vi "PH_PILS.set Doors Beam Diag.vi"(0 "i ref in":refnum<vi>, 2 "Service Name":string="N/A", 5 "error in":errorcluster) -> (14 "i ref out":refnum<vi>, 19 "error out":errorcluster)   [LabVIEW 2014, in "PH_PILS.lvlib"]
doc: "This VI sets the GUI elements related to the doors at the beam Diagnostic."
uses:
  PH_PILS.lvlib
  PH_PILS.Operation Mode.ctl
  PH_Common/PH_Common.lvlib
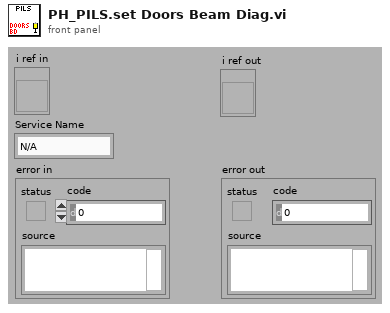
[diagram p1: front panel]
types:
  T1 = typedef "PH_PILS.lvlib/PH_PILS.Operation Mode.ctl" = enum16{"unknown", "Service", "Labor", "Search", "Shot"}
  T2 = typedef "PH_PILS.lvlib/PH_PILS.i attribute.ctl" = cluster{"Boolean":cluster{"GUI Ref":refnum<vi>, "Status":i32}[], "GUI Refs Exp. Shutters":cluster{"1":refnum<vi>, "2":refnum<vi>, "3":refnum<vi>, "4":refnum<vi>}, "Tristate2Run GUI Refs":refnum<vi>[], "EO-Likes":cluster{"GUI Ref":refnum<vi>, "Status":i32}[], "Operation Mode":cluster{"Operation Mode":T1, "GUI":cluster{"Ref State":refnum<vi>, "Ref":refnum<vi>}, "Servicemode":cluster{"Tagname":string, "Status":i32}, "Labormode":cluster{"Tagname":string, "Status":i32}, "Searchmode":cluster{"Tagname":string, "Status":i32}, "Shotmode":cluster{"Tagname":string, "Status":i32}}, "Submode":cluster{"Submode":T3, "GUI":cluster{"Ref State":refnum<vi>, "Ref":refnum<vi>}, "Submode":cluster{"Tagname":string, "Status":i32}}, "Experiment":cluster{"Experiment":enum16{"unknown", "intern", "4 (Z6)", "3", "2", "1"}, "GUI":cluster{"Ref State":refnum<vi>, "Ref":refnum<vi>}, "intern":cluster{"Tagname":string, "Status":i32}, "Exp 4":cluster{"Tagname":string, "Status":i32}, "Exp 3":cluster{"Tagname":string, "Status":i32}, "Exp 2":cluster{"Tagname":string, "Status":i32}, "Exp 1":cluster{"Tagname":string, "Status":i32}}, "TristateNormal":cluster{"GUI Ref":refnum<vi>, "Status":i32}[], "Door Tags":cluster{"GUI Ref":refnum<vi>, "Status":i32}[], "GUIlessTags":cluster{"Name":string, "Status":i32}[], "Beamline GUI Refs":refnum<vi>[], "Special Boolean":cluster{"GUI Ref":refnum<vi>, "Status":i32}[], "Laserpower":cluster{"GUI Ref":refnum<vi>, "Status":i32}[], "Shutter":cluster{"GUI Ref":refnum<vi>, "Status":i32}[], "Tristate EO Like":cluster{"GUI Ref":refnum<vi>, "Status":i32}[], "PP":cluster{"GUI Ref":refnum<vi>, "Status":i32, "Head Ref":refnum<vi>, "Slider Ref":refnum<vi>}[], "Switch Knobs":cluster{"GUI Ref":refnum<vi>, "Status":i32}[], "Latch Knob GUI Refs":refnum<vi>[], "FailureCounter":i32, "Enabled Status":cluster{"Laser":i32, "PreAmp":i32, "MainAmp":i32}, "Mercury":refnum<vi>, "Instance Rods":string, "Logfile":path, "Beckhoff-Instance Internal":string, "Beckhoff-Instance External":string, "Enabling Rights":cluster{"Name":string, "Password":string, "PA?":bool, "MA?":bool, "Exp?":bool}[]}
  T3 = typedef "PH_PILS.lvlib/PH_PILS.Submode.ctl" = enum16{"unknown", "HV-Normal", "HV-Test"}
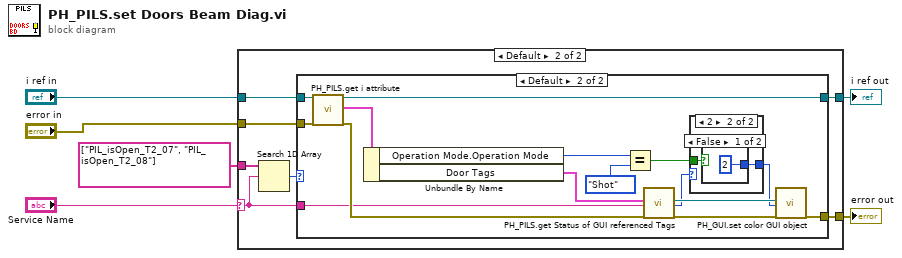
[diagram p0: block diagram]
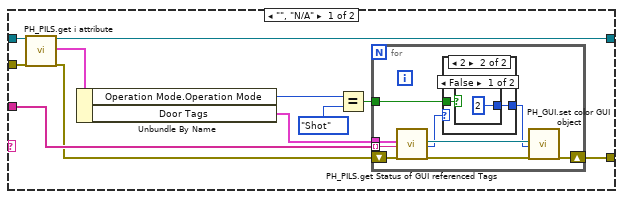
[diagram p2: hidden frame]
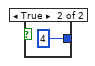
[diagram p4: hidden frame]
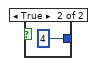
[diagram p7: hidden frame]
diagram:
  n1 = case shown="Default" "Service Name" {
    selector: "Service Name" -> [_ w34]
    tunnel: "error in" -> [w17 w38]
    tunnel: [w16 w37] -> w5
    tunnel: "i ref in" -> [w15 w36]
    tunnel: [w13 w35] -> w3
    tunnel: string[] ["PIL_isOpen_T2_07", "PIL_isOpen_T2_08"] -> [w12 w33]
    frame "", "N/A" {
      n2 = call "PH_PILS.get i attribute.vi"("i ref in"=w15, "error in (no error)"=w17) -> ("i ref out"=w16:refnum<vi>, "i attribute"=w14:T2, "error out"=w7:errorcluster)  [unwired: 15 in]
      n3 = Unbundle By Name(w14) -> ("Operation Mode.Operation Mode"=w11:T1, "Door Tags"=w8:cluster{"GUI Ref":refnum<vi>, "Status":i32}[])
      n4 = Equal?(x=w11, y=PH_PILS.Operation_Mode."Shot" ("Operation Mode.Operation Mode")) -> (x = y?=w9:bool)
      n5 = for {
        tunnel: w8 -> [w26]
        tunnel: w12 -> [w23] mode=indexing
        shift-right: [w22] -> w13
        shift-left: w7 -> [w25]
        tunnel: w9 -> [w18]
        n6 = call "PH_PILS.get Status of GUI referenced Tags.vi"("Tags"=w26, "Tagname"=w23, "error in"=w25) -> ("GUI Ref"=w21:refnum<vi>, "Status"=w20:i32, "error out"=w24:errorcluster)  [unwired: 13 in, 1 out]
        n7 = case shown="2" w20 {
          selector: w20 -> [w27 _]
          tunnel: [w27 w29] -> w19
          tunnel: w18 -> [_ w28]
          frame 0, Default {
          }
          frame 2 {
            n8 = case shown="False" w28 {
              tunnel: [2 4] -> w29
              frame False {
              }
              frame True {
              }
            }
          }
        }
        n9 = call "PH_GUI.set color GUI object.vi"("GUI object Ref"=w21, "State"=w19, "error in (no error)"=w24) -> ("error out"=w22:errorcluster)  [unwired: 16 in]
      }
    }
    frame Default {
      n10 = Search 1D Array(1D array=w33, element=w34) -> (index of element=w32:i32)  [unwired: 1 in]
      n11 = case shown="Default" w32 {
        tunnel: w38 -> [w39 w55]
        tunnel: [w40 w54] -> w37
        tunnel: w36 -> [w40 w53]
        tunnel: [w39 w51] -> w35
        tunnel: w34 -> [_ w45]
        frame -1 {
        }
        frame Default {
          n12 = call "PH_PILS.get i attribute.vi"("i ref in"=w53, "error in (no error)"=w55) -> ("i ref out"=w54:refnum<vi>, "i attribute"=w52:T2, "error out"=w46:errorcluster)  [unwired: 15 in]
          n13 = Unbundle By Name(w52) -> ("Operation Mode.Operation Mode"=w50:T1, "Door Tags"=w47:cluster{"GUI Ref":refnum<vi>, "Status":i32}[])
          n14 = Equal?(x=w50, y=PH_PILS.Operation_Mode."Shot" ("Operation Mode.Operation Mode")) -> (x = y?=w48:bool)
          n15 = call "PH_PILS.get Status of GUI referenced Tags.vi"("Tags"=w47, "Tagname"=w45, "error in"=w46) -> ("GUI Ref"=w43:refnum<vi>, "Status"=w42:i32, "error out"=w44:errorcluster)  [unwired: 13 in, 1 out]
          n16 = case shown="2" w42 {
            selector: w42 -> [w56 _]
            tunnel: [w56 w58] -> w41
            tunnel: w48 -> [_ w57]
            frame 0, Default {
            }
            frame 2 {
              n17 = case shown="False" w57 {
                tunnel: [2 4] -> w58
                frame False {
                }
                frame True {
                }
              }
            }
          }
          n18 = call "PH_GUI.set color GUI object.vi"("GUI object Ref"=w43, "State"=w41, "error in (no error)"=w44) -> ("error out"=w51:errorcluster)  [unwired: 16 in]
        }
      }
    }
  }
  "error out" <- w3
  "i ref out" <- w5
